vi "init_logs.vi"(8 "error in (no error)":errorcluster, 11 "Cluster":T1) -> (0 "error out":errorcluster, 3 "Cluster out":T1)   [LabVIEW 2024, in "Download_Manager.lvlib"]
uses:
  Download_Manager.lvlib
  <vilib>/addons/_JKI.lib/REST Client/classes/REST Client/REST Client.lvclass
  typedefs/job--cluster.ctl
  typedefs/job_type--enum.ctl
  comic_manager/manager_daemon/manager_daemon.lvclass
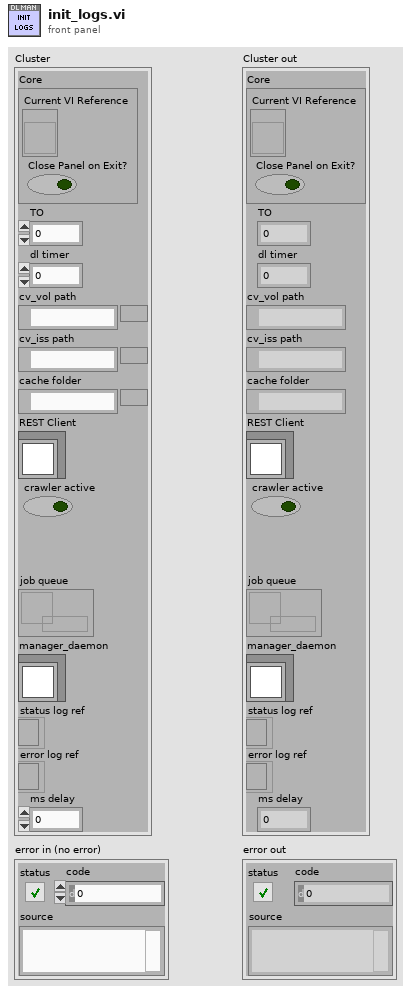
[diagram p1: front panel]
types:
  T1 = cluster{"Core":cluster{"Current VI Reference":refnum<vi>, "Close Panel on Exit?":bool}, "TO":i32, "dl timer":u32, "cv_vol path":path, "cv_iss path":path, "cache folder":path, "REST Client":refnum<class "REST Client.lvclass">, "crawler active":bool, "job queue":refnum<queue>, "manager_daemon":refnum<class "manager_daemon.lvclass">, "status log ref":refnum<file>, "error log ref":refnum<file>, "ms delay":u32}
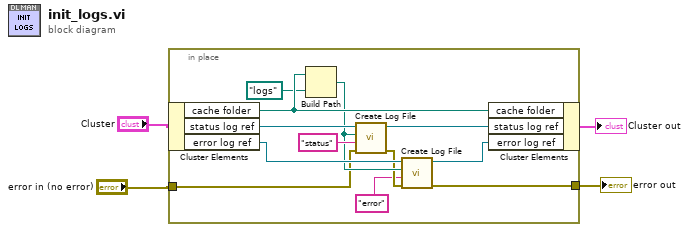
[diagram p0: block diagram]
diagram:
  n1 = in-place {
    in-place-border: [w7] -> w2
    in-place-border: "error in (no error)" -> [w6]
    n2 = in-place-cluster #1("Cluster") -> ("cache folder"=w14:path, "status log ref"=w16:refnum<file>, "error log ref"=w10:refnum<file>)
    n3 = Build Path(base path=w14, name or relative path=path "logs") -> (appended path=w9:path)
    n4 = call "Create Log File.vi"("error in (no error)"=w6, "name prefix"="status", "Directory"=w9, "file reference in"=w16) -> ("error out"=w8:errorcluster, "file reference out"=w15:refnum<file>)  [unwired: 6 in]
    n5 = call "Create Log File.vi"("error in (no error)"=w8, "name prefix"="error", "Directory"=w9, "file reference in"=w10) -> ("error out"=w7:errorcluster, "file reference out"=w11:refnum<file>)  [unwired: 6 in]
    n6 = in-place-cluster #1("cache folder"=w14, "status log ref"=w15, "error log ref"=w11) -> (→"Cluster out":T1)
  }
  "error out" <- w2
